vi "Test Base Error Flow Through.vi"(8 "error in (no error)":errorcluster, 11 "Base Class Test In":refnum<class "Base Test.lvclass">) -> (0 "error out":errorcluster, 3 "Base Class Test Out":refnum<class "Base Test.lvclass">)   [LabVIEW 2020, in "Base Test.lvclass"]
uses:
  Base Test.lvclass
  C:/Program Files (x86)/National Instruments/LabVIEW 2020/vi.lib/Astemes/LUnit/Test Case.lvclass
  Base Test.lvclass/Base Test.ctl
  <vilib>/Astemes/LUnit/Test Case.lvclass/Test Case.ctl
  <vilib>/Astemes/LUnit/LUnit Assertion Result.lvclass/LUnit Assertion Result.ctl
  <vilib>/Astemes/LUnit/LUnit Test Case Result.lvclass/LUnit Test Case Result.ctl
  <vilib>/Astemes/LUnit/LUnit Method Result.lvclass/LUnit Method Result.ctl
  cbbbb4fa-fbe2-4001-b1af-9e48cfedae24.vi
  <vilib>/Astemes/LUnit/Palette/Pass.vi
  <vilib>/Astemes/LUnit/Palette/Fail.vi
  <vilib>/Astemes/LUnit/Compare Variants.vi
  <vilib>/Astemes/LUnit/Describe Comparison.vi
  <vilib>/Astemes/LUnit/Set Assertion Type.vi
  <vilib>/Astemes/LUnit/Add test result.vi
  <vilib>/Astemes/LUnit/LUnit Write Passed.vi
  <vilib>/Astemes/LUnit/LUnit Write Message.vi
  <vilib>/Astemes/LUnit/LUnit Write Description.vi
  <vilib>/Astemes/LUnit/Variant to string.vi
  <vilib>/Astemes/LUnit/LUnit Write Assertion Type.vi
  <vilib>/Astemes/LUnit/LUnit Record Assertion Result.vi
  <vilib>/Astemes/LUnit/LUnit Aggregate Assertion Results.vi
  <vilib>/Astemes/LUnit/Assertion Result/LUnit Read Status.vi
  <vilib>/Astemes/LUnit/LUnit Read Message.vi
  <vilib>/Astemes/LUnit/LUnit Read Description.vi
  <vilib>/Astemes/LUnit/Method Result/LUnit Merge Status.vi
  <vilib>/Astemes/LUnit/LUnit Concatenate result strings.vi
  <vilib>/Utility/error.llb/Error Cluster From Error Code.vi
  <vilib>/Utility/Data Type/Get Type Information.vi
  <vilib>/Utility/LVClass/Get LV Class Name.vi
  Framework/Base/Base.lvclass
  <vilib>/ErrorRing/Error Ring.xnode
  <vilib>/Astemes/LUnit/LUnit Assertion Result.lvclass
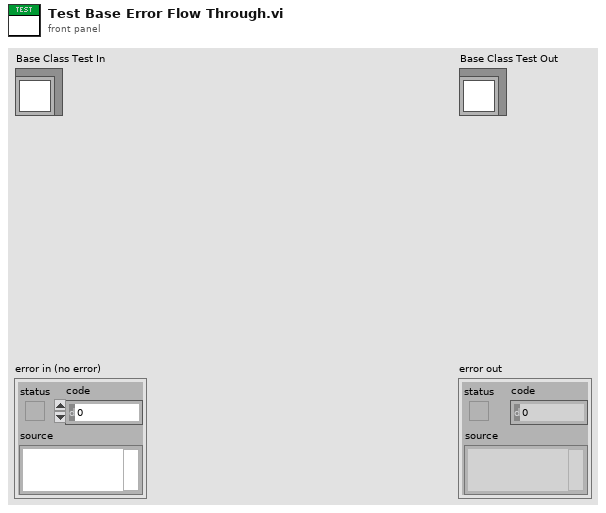
[diagram p1: front panel]
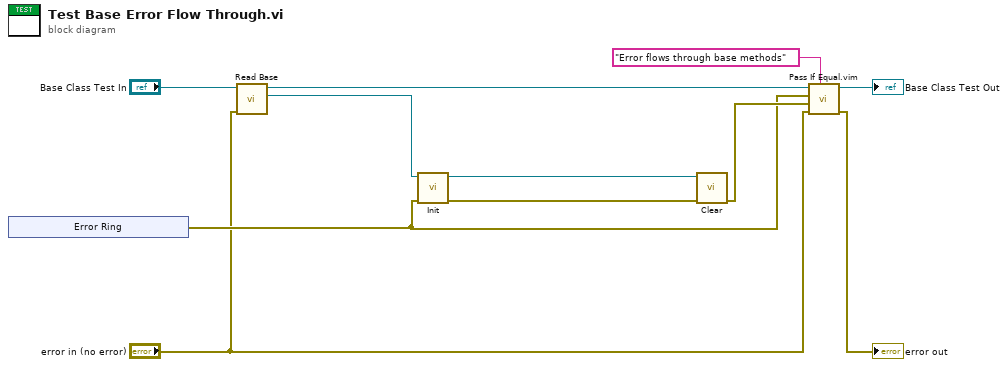
[diagram p0: block diagram]
diagram:
  n1 = xnode "Error Ring"() -> ("error out"=w4:errorcluster)
  n2 = call "Read Base.vi"("error in (no error)"="error in (no error)", "Base Class Test In"="Base Class Test In") -> ("Base.lvclass"=w7:refnum<class "Base.lvclass">, "Base Class Test Out"=w10:refnum<class "Base Test.lvclass">)  [unwired: 7 in, 1 out]
  n3 = call-dynamic "Init.vi"("error in (no error)"=w4, "Base In"=w7) -> ("error out"=w8:errorcluster, "Base Out"=w9:refnum<class "Base.lvclass">)  [unwired: 8 in]
  n4 = call-dynamic "Clear.vi"("error in (no error)"=w8, "Base In"=w9) -> ("error out"=w5:errorcluster)  [unwired: 9 in]
  n5 = call "Pass If Equal.vim"("Description"="Error flows through base methods", "error in (no error)"="error in (no error)", "Actual"=w5, "Expected"=w4, "LUnit Test Case In"=w10) -> ("error out"=→"error out":errorcluster, "LUnit Test Case Out"=→"Base Class Test Out":refnum<class "Base Test.lvclass">)  [unwired: 5 in]
